vi "spectral_map.vi"(6 "YEND":i16=300, 8 "XEND":i16=300, 9 "YSTART":i16=1, 10 "XSTART":i16=1, 11 "Path_image":path=path "C:/Users/swift/Desktop/Python/imec/Data/SKFX.300x300.Binning.2.frame.1.Gain.1.time.5.HDR-V6_corrected.hdr") -> ()   [LabVIEW 2018]
panel:
  out "Image":T1(plugin-control)
  out "size(s)":i32[](array[numeric])
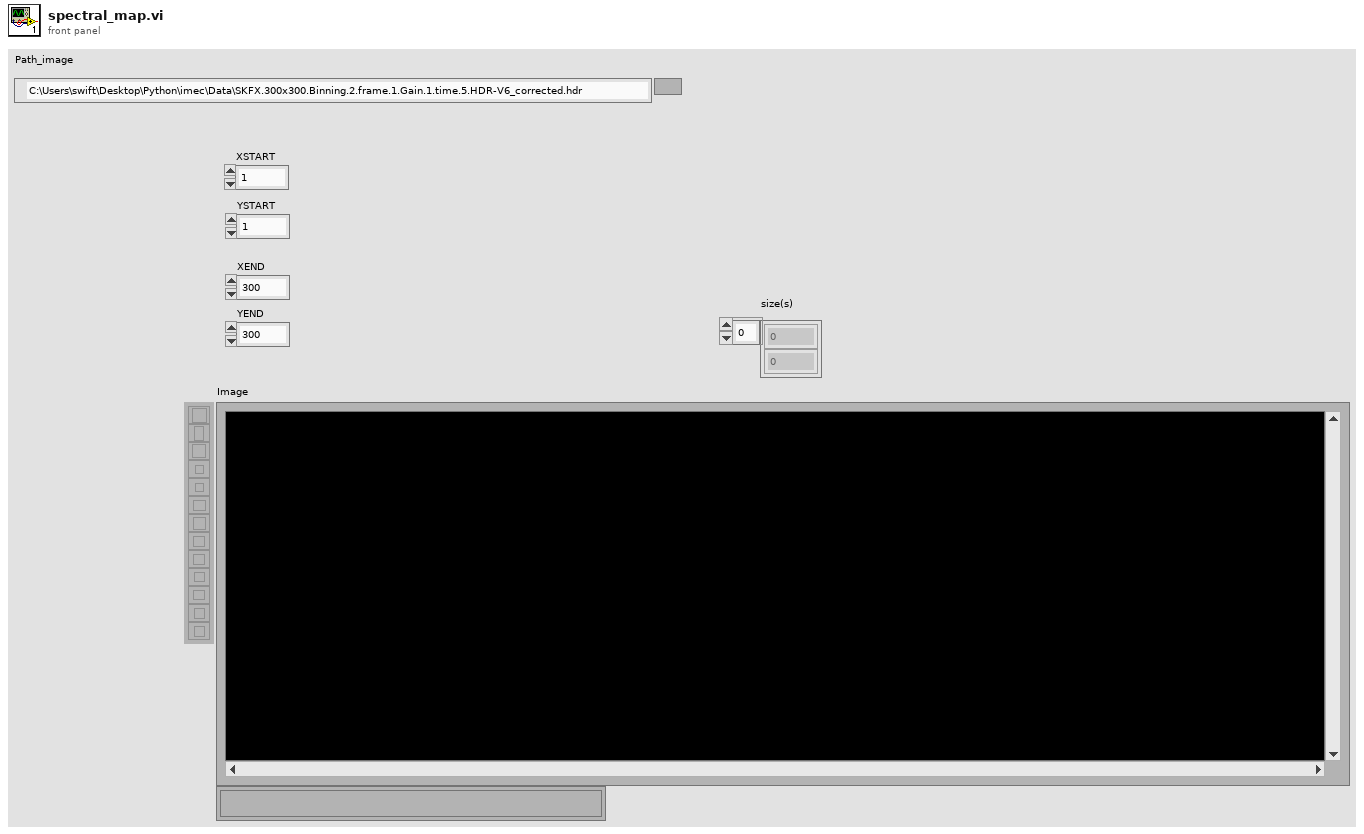
[diagram p1: front panel]
types:
  T1 = typedef "IMAQ Image.ctl" = refnum<image>
  T2 = typedef "Image Type" = u32
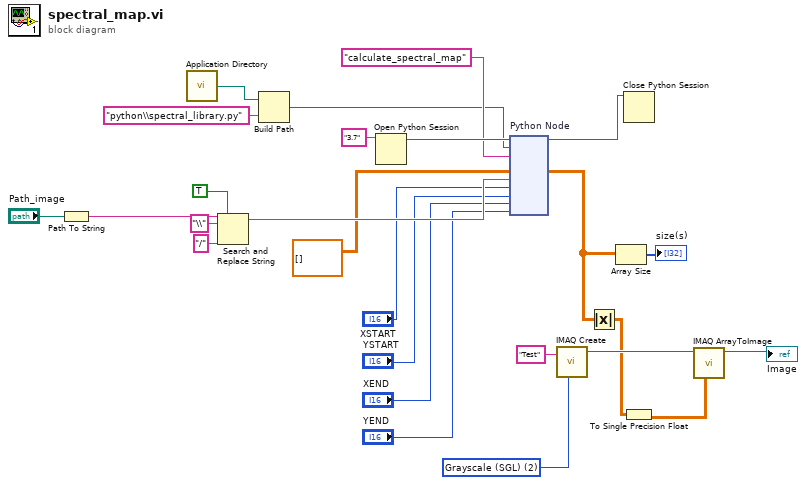
[diagram p0: block diagram]
diagram:
  w3 = T2 2 items=["Grayscale (U8)", "Grayscale (I16)", "Grayscale (SGL)", "Complex (CSG)", "RGB (U32)", "HSL (U32)", "RGB (U64)", "Grayscale (U16)"] ("Image Type")
  n1 = Path To String(path="Path_image") -> (string=w18:string)
  n2 = call <vilib>:"Application Directory.vi"() -> ("Application Directory"=w23:path)
  n3 = Search and Replace String(replace all?=TRUE ("replace all? (F)"), input string=w18, search string="\\", replace string="/" ("replace string (\"\")")) -> (result string=w14:string)  [unwired: 4 in, 3 out]
  n4 = Build Path(base path=w23, name or relative path="python\\spectral_library.py" ("nom ou chemin relatif")) -> (appended path=w21:path)
  n5 = Open Python Session(python version="3.7" ("Python version")) -> (session out=w25:refnum<k35>)  [unwired: 2 in, 1 out]
  n6 = node "Python Node"(w25, w21, "calculate_spectral_map" ("function name"), dbl[][] [], w14, "XSTART", "YSTART", "XEND", "YEND") -> (w20:refnum<k35>, w7:dbl[][])  [unwired: 6 in, 3 out]
  n7 = call "IMAQ Create"("Image Name"="Test", "Image Type"=w3) -> ("New Image"=w6:T1)  [unwired: 3 in, 1 out]
  n8 = Absolute Value(x=w7) -> (abs(x)=w4:dbl[][])
  n9 = Array Size(array=w7) -> (size(s)=→"size(s)":i32[])
  n10 = Close Python Session(session in=w20) -> ()  [unwired: 1 in, 1 out]
  n11 = To Single Precision Float(number=w4) -> (single precision float=w1:sgl[][])
  n12 = call "IMAQ ArrayToImage"("Image Pixels (Float)"=w1, "Image"=w6) -> ("Image Out"=→"Image":T1)  [unwired: 8 in, 1 out]
